vi "电流采样测试与校准.vi"(0 "仪器实例 in":T1, 2 "?":dbl[](array[numeric]), 3 "error in":errorcluster caption="错误输入") -> (6 "总判定":bool, 7 "仪器实例 out":T1, 8 "测试结果":cluster{"测试结果":dbl[][], "斜率":dbl, "截距":dbl}, 9 "判定数组":bool[](array[boolean]), 10 "error out":errorcluster caption="错误输出")   [LabVIEW 2020]
uses:
  F:/F020/S7_1200 control/HslCommunication.dll
  S7_1200 control/HslCommunication.dll
panel:
  in  "误差":dbl=0.005 format="%#_13g"
  in  "簇":cluster{"产品条码":string, "分流器条码":string}
  out "表格控件":string[][](table) caption="测试结果"
  # "F020 分流器标定测试系统"
  # "仪器地址设置"
  # "产品信息"
  # "电流条件"
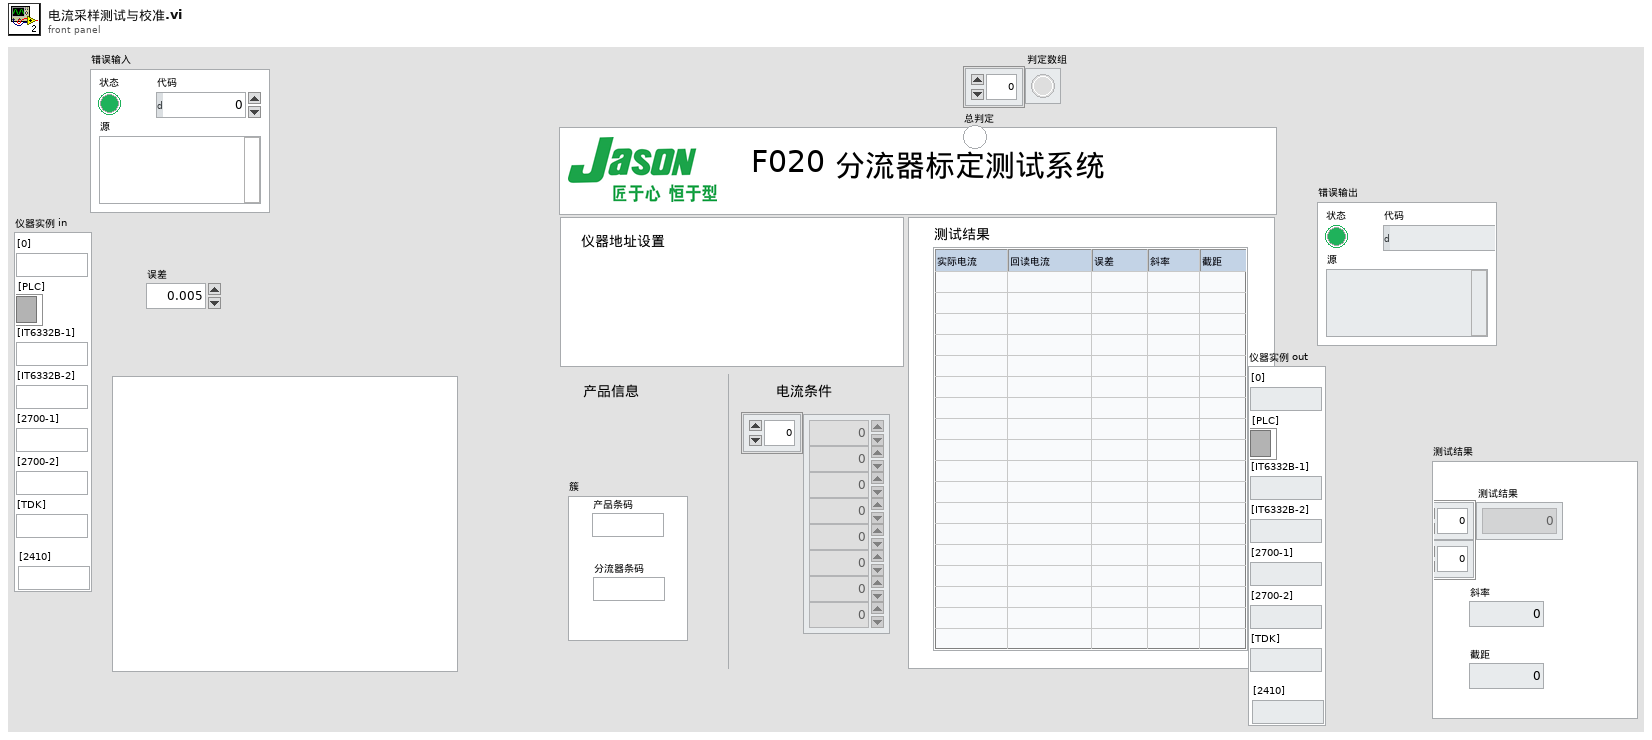
[diagram p1: front panel]
types:
  T1 = typedef "仪器实例.ctl" = cluster{"[0]":string, "[PLC]":refnum<k24>, "[IT6332B-1]":string, "[IT6332B-2]":string, "[2700-1]":string, "[2700-2]":string, "[TDK]":string, "[2410]":string}
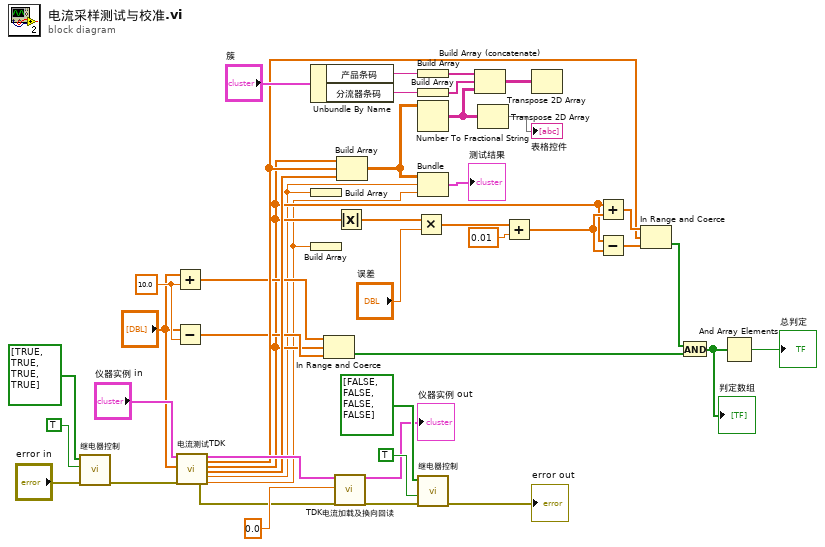
[diagram p0: block diagram]
diagram:
  w13 = 10.0
  n1 = call "继电器控制.vi"("error in"="error in", "初始化"=TRUE, "继电器控制"=bool[] [TRUE, TRUE, TRUE, TRUE]) -> ("error out"=w36:errorcluster)  [unwired: 8 in]
  n2 = Add(x="?", y=w13) -> (x+y=w10:dbl[])
  n3 = Subtract(x="?", y=w13) -> (x-y=w11:dbl[])
  n4 = call "电流测试TDK.vi"("仪器实例 in"="仪器实例 in", "电流测试点"="?", "error in (no error)"=w36) -> ("error out"=w34:errorcluster, "仪器实例 out"=w33:T1, "回读电流"=w14:dbl[], "输入电流"=w9:dbl[], "误差"=w15:dbl[], "斜率"=w2:dbl, "截距"=w3:dbl)  [unwired: 10 in]
  n5 = Unbundle By Name("簇") -> ("产品条码"=w26:string, "分流器条码"=w25:string)
  n6 = Build Array(w2) -> ()  [unwired: 1 out]
  n7 = Build Array(w3) -> ()  [unwired: 1 out]
  n8 = In Range and Coerce(upper limit=w10, x=w9, lower limit=w11) -> (In Range?=w8:bool[])  [unwired: 1 out]
  n9 = call "TDK电流加载及换向回读.vi"("仪器实例 in"=w33, "输入电流"=0.0, "error in"=w34) -> ("仪器实例 out"=→"仪器实例 out":T1, "error out"=w32:errorcluster)  [unwired: 14 in, 1 out]
  n10 = Absolute Value(x=w9) -> (abs(x)=w19:dbl[])
  n11 = Build Array(w9, w14, w15) -> (w4:dbl[][])
  n12 = Multiply(x=w19, y="误差") -> (x*y=w20:dbl[])
  n13 = Build Array(w26) -> (w43:string[])
  n14 = Build Array(w25) -> (w42:string[])
  n15 = Number To Fractional String(number=w4) -> (F-format string=w40:string[][])  [unwired: 3 in]
  n16 = Bundle(w4, "斜率"=w2, "截距"=w3) -> (→"测试结果":cluster{dbl[][], "斜率":dbl, "截距":dbl})  [unwired: 1 in]
  n17 = call "继电器控制.vi"("error in"=w32, "释放"=TRUE, "继电器控制"=bool[] [FALSE, FALSE, FALSE, FALSE]) -> ("error out"=→"error out":errorcluster)  [unwired: 8 in]
  n18 = Build Array (concatenate)(w43, w42, w40) -> (w41:string[][])
  n19 = Transpose 2D Array(2D array=w40) -> (transposed array=→"表格控件":string[][])
  n20 = Add(x=w20, y=0.01) -> (x+y=w17:dbl[])
  n21 = Transpose 2D Array(2D array=w41) -> ()  [unwired: 1 out]
  n22 = Add(x=w9, y=w17) -> (x+y=w18:dbl[])
  n23 = Subtract(x=w9, y=w17) -> (x-y=w16:dbl[])
  n24 = In Range and Coerce(upper limit=w18, x=w14, lower limit=w16) -> (In Range?=w7:bool[])  [unwired: 1 out]
  n25 = And(x=w7, y=w8) -> (x .and. y?=w6:bool[])
  "判定数组" <- w6
  n26 = And Array Elements(Boolean array=w6) -> (logical AND=→"总判定":bool)
